vi "subVI Read Excel file into array.vi"(10 "Select row & col to read":T1, 11 "Filepath":path[](array[path])=[path "C:/Users/Main User/Desktop/Research/Cocktail maker/LABVIEW/LabVIEW Paper Automation/LabVIEW Test for modularizing program/SequenceProgram.xlsx"]) -> (2 "1D vector output":dbl[](array[numeric]), 3 "2D matrix output":dbl[][](array[numeric]))   [LabVIEW 2019]
panel:
  out "3D data read-out":dbl[][][](array[numeric])
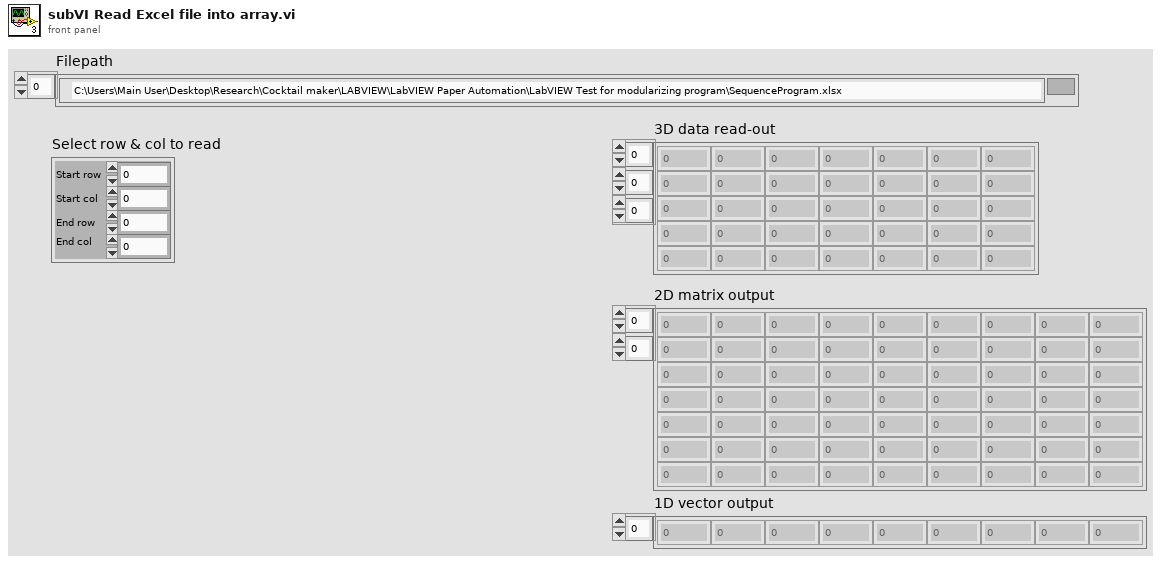
[diagram p1: front panel]
types:
  T1 = cluster{"Start row":i32, "Start col":i32, "End row":i32, "End col":i32}
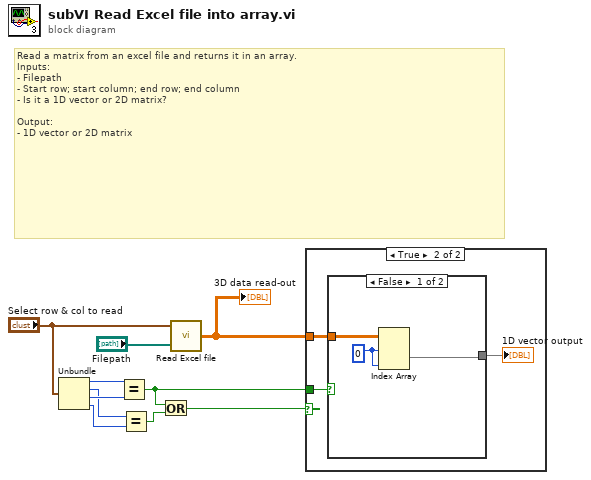
[diagram p0: block diagram]
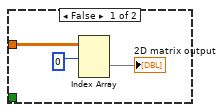
[diagram p2: hidden frame]
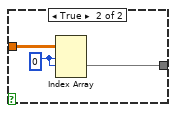
[diagram p3: hidden frame]
diagram:
  # "Read a matrix from an excel file and returns it in an array.\nInputs:\n- Filepath\n- Start row; start column; end row; end column\n- Is it a 1D vector or 2D matrix?\n\nOutput:\n- 1D vector or 2D matrix"
  n1 = Unbundle("Select row & col to read") -> ("Start row"=w8:i32, "Start col"=w5:i32, "End row"=w7:i32, "End col"=w4:i32)
  n2 = Equal?(x=w8, y=w7) -> (x = y?=w1:bool)
  n3 = Equal?(x=w5, y=w4) -> (x = y?=w6:bool)
  n4 = Or(x=w1, y=w6) -> (x .or. y?=w3:bool)
  n5 = call "Read Excel file.vi"("Array"="Filepath", "Start and End"="Select row & col to read") -> ("array"=w2:dbl[][][])
  "3D data read-out" <- w2
  n6 = case shown="True" w3 {
    tunnel: w2 -> [w11 w15]
    tunnel: w1 -> [_ w16]
    frame False {
      n7 = Index Array(array=w11, index (dim 0)=0 ("disabled index (col) 2")) -> (element=→"2D matrix output":dbl[][])  [unwired: 2 in]
    }
    frame True {
      n8 = case shown="False" w16 {
        tunnel: w15 -> [w19 w21]
        tunnel: [w17 w20] -> w14
        frame False {
          w18 = 0 ("disabled index (col) 2")
          n9 = Index Array(array=w19, index (dim 0)=w18, index (dim 2)=w18) -> (element=w17:dbl[])  [unwired: 1 in]
        }
        frame True {
          w22 = 0 ("disabled index (col) 2")
          n10 = Index Array(array=w21, index (dim 0)=w22, index (dim 1)=w22) -> (element=w20:dbl[])  [unwired: 1 in]
        }
      }
      "1D vector output" <- w14
    }
  }
